vi "ErrorTransmitter.vi"(8 "Error In":errorcluster) -> (0 "Error Out":errorcluster)   [LabVIEW 2013]
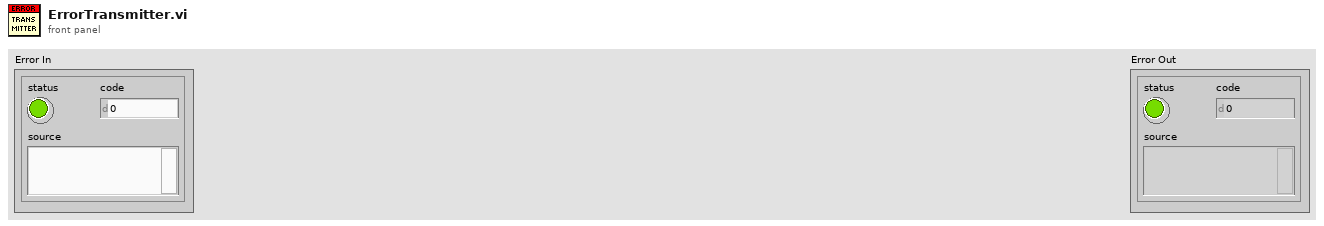
[diagram p1: front panel]
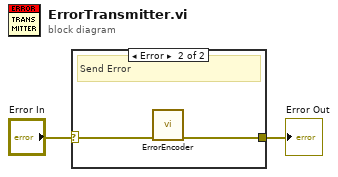
[diagram p0: block diagram]
diagram:
  n1 = case shown="Error" "Error In" {
    selector: "Error In" -> [w3 w5]
    tunnel: [w3 w4] -> w1
    frame No Error {
      # "No Error"
    }
    frame Error {
      # "Send Error"
      n2 = call "ErrorEncoder.vi"("Error In"=w5) -> ("Error Out"=w4:errorcluster)  [unwired: 10 in]
    }
  }
  "Error Out" <- w1
